vi "Get Capacity.vi"(8 "error in (no error)":errorcluster, 11 "VISA resource name":refnum<visa-resource-name>) -> (0 "error out":errorcluster, 1 "Capacity (out)":i8, 3 "VISA resource name out":refnum<visa-resource-name>)   [LabVIEW 2018, in "JULABO DeviceDriver.lvlib"]
doc: "This VI returns the actual heating or cooling capacity"
uses:
  JULABO DeviceDriver.lvlib
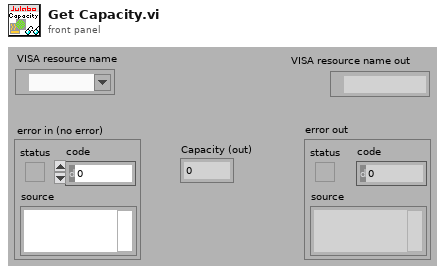
[diagram p1: front panel]
types:
  T1 = typedef "JULABO DeviceDriver.lvlib/InstrumentType.ctl" = enum8{"Default", "FC-Series", "HT30/HT60", "LC4"}
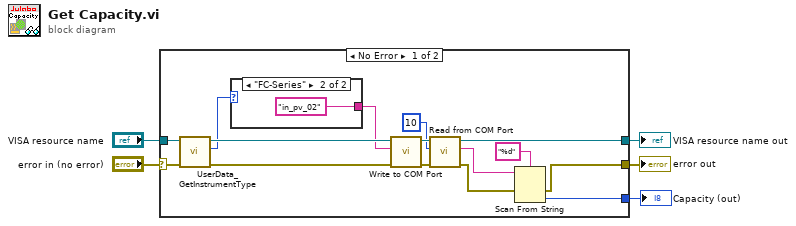
[diagram p0: block diagram]
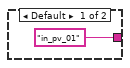
[diagram p2: hidden frame]
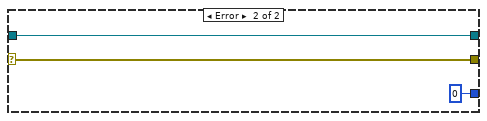
[diagram p3: hidden frame]
diagram:
  n1 = case shown="No Error" "error in (no error)" {
    selector: "error in (no error)" -> [w11 w24]
    tunnel: "VISA resource name" -> [w10 w25]
    tunnel: [w15 w24] -> w4
    tunnel: [w14 w25] -> w3
    tunnel: [w12 0] -> w2
    frame No Error {
      n2 = call "UserData_GetInstrumentType.vi"("Fehler (Eingang)"=w11, "VISA resource name in"=w10) -> ("Fehler (Ausgang)"=w8:errorcluster, "InstrumentType"=w7:T1, "VISA resource name out"=w9:refnum<visa-resource-name>)  [unwired: 3 in]
      n3 = case shown="\"FC-Series\"" w7 {
        tunnel: ["in_pv_01" "in_pv_02"] -> w6
        frame Default {
        }
        frame "FC-Series" {
        }
      }
      n4 = call "Write to COM Port.vi"("error in"=w8, "Command (input)"=w6, "VISA resource name in"=w9) -> ("error out"=w20:errorcluster, "VISA resource name out"=w19:refnum<visa-resource-name>)  [unwired: 7 in]
      n5 = call "Read from COM Port.vi"("error in"=w20, "Byte to Read (-1:All)"=u32 10 ("Anzahl der Byte"), "VISA resource name in"=w19) -> ("error out"=w17:errorcluster, "String (output)"=w16:string, "VISA resource name out"=w14:refnum<visa-resource-name>)  [unwired: 5 in, 1 out]
      n6 = Scan From String(format string="%d" ("Format-String"), input string=w16, error in=w17) -> (error out=w15:errorcluster, output 1=w12:i32)  [unwired: 2 in, 2 out]
    }
    frame Error {
    }
  }
  "error out" <- w4
  "VISA resource name out" <- w3
  "Capacity (out)" <- w2
